vi "SQL_UploadMachines.vi"   [LabVIEW 2017]
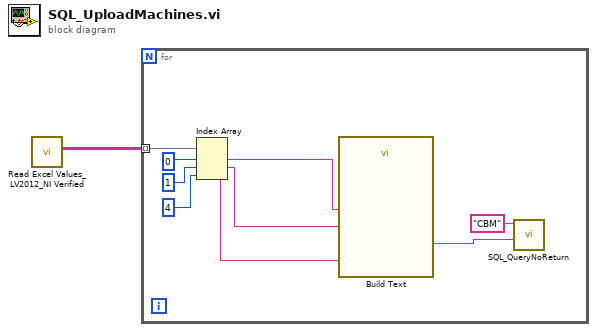
[diagram p0: block diagram]
diagram:
  n1 = call "Read Excel Values_LV2012_NI Verified.vi"() -> ("ExcelData"=w1:string[][])  [unwired: 11 in]
  n2 = for {
    tunnel: w1 -> [w10] mode=indexing
    n3 = Index Array(array=w10, index #1=0, index #2=1, index #3=4) -> (element #1=w7:string, element #2=w6:string, element #3=w2:string)
    n4 = call "Build Text"("toolcribpn"=w7, "description"=w6, "location"=w2) -> ("Result"=w5:string)  [unwired: 11 in, 1 out]
    n5 = call "SQL_QueryNoReturn.vi"("SQL query"=w5, "ConnectionDSN"="CBM") -> ()  [unwired: 10 in]
  }
